vi "Test App Trigger Broadcast of Owned Process.vi"(8 "error in (no error)":errorcluster, 11 "Application Test in":refnum<class "Application Dev Test.lvclass">) -> (0 "error out":errorcluster, 3 "Application Test out":refnum<class "Application Dev Test.lvclass">)   [LabVIEW 2020, in "Application Dev Test.lvclass"]
uses:
  Application Dev Test.lvclass
  C:/Program Files (x86)/National Instruments/LabVIEW 2020/vi.lib/Astemes/LUnit/Test Case.lvclass
  source/Framework/Process/Process.lvclass
  source/Framework/Process/Process.lvclass/Process.ctl
  source/Framework/Application/Application.lvclass/Application.ctl
  <vilib>/Astemes/LUnit/Test Case.lvclass/Test Case.ctl
  <vilib>/Astemes/LUnit/LUnit Assertion Result.lvclass/LUnit Assertion Result.ctl
  <vilib>/Astemes/LUnit/LUnit Test Case Result.lvclass/LUnit Test Case Result.ctl
  <vilib>/Astemes/LUnit/LUnit Method Result.lvclass/LUnit Method Result.ctl
  source/Framework/Application/Private/Add Process to Map.vi
  source/Framework/Application/Private/Start Idle Processes if Running.vi
  source/Framework/Application/Private/Throw Error If Process Already in App.vi
  source/Framework/Process/Protected/Messaging/Enqueue Message.vi
  source/Framework/Process/Public/Lifecycle/Get Lifecycle State.vi
  source/Framework/Process/Protected/SubVIs/Set Context.vi
  source/Framework/Process/Private/SubVIs/Wait for finish.vi
  source/Framework/Process/Private/SubVIs/Set Lifecycle State.vi
  <vilib>/Astemes/LUnit/Palette/Fail.vi
  <vilib>/Astemes/LUnit/Palette/Pass.vi
  <vilib>/Astemes/LUnit/Set Assertion Type.vi
  source/Framework/Application/Public/Get Process.vi
  source/Framework/Process/Private/SubVIs/Handle Debug Data.vi
  <vilib>/Utility/error.llb/Clear Errors.vi
  source/Framework/Process/Public/Lifecycle/Leave Process Loop.vi
  <vilib>/Astemes/LUnit/Add test result.vi
  <vilib>/Astemes/LUnit/LUnit Write Passed.vi
  <vilib>/Astemes/LUnit/LUnit Write Message.vi
  <vilib>/Astemes/LUnit/LUnit Write Description.vi
  <vilib>/Astemes/LUnit/LUnit Write Assertion Type.vi
  source/Framework/Application/Private/Retrieve Process from App.vi
  source/Framework/Application/Private/Parse Process Name.vi
  source/Framework/Application/Private/Get Process from Map.vi
  source/Framework/Logging/Log Debug.vi
  <vilib>/AdvancedString/1D String Array to Delimited String.vi
  <vilib>/Utility/High Resolution Relative Seconds.vi
  <vilib>/Astemes/LUnit/LUnit Record Assertion Result.vi
  source/Framework/Process/Protected/Messaging/Request Message.vi
  <vilib>/AdvancedString/Delimited String to 1D String Array.vi
  <vilib>/Astemes/LUnit/LUnit Aggregate Assertion Results.vi
  source/Framework/Process/Private/SubVIs/Enqueue Request Message.vi
  <vilib>/Astemes/LUnit/Assertion Result/LUnit Read Status.vi
  <vilib>/Astemes/LUnit/LUnit Read Message.vi
  <vilib>/Astemes/LUnit/LUnit Read Description.vi
  <vilib>/Astemes/LUnit/Method Result/LUnit Merge Status.vi
  <vilib>/Astemes/LUnit/LUnit Concatenate result strings.vi
  source/Framework/Application/Application.lvclass
  C:/Git/astemes-triarc-framework/source/Framework/Process/Process.lvclass
  <vilib>/Utility/error.llb/Error Cluster From Error Code.vi
  source/Framework/Process/Public/Read Name.vi
  source/Framework/Process/Private/SubVIs/Wait for Response Message.vi
  <vilib>/Astemes/LUnit/LUnit Assertion Result.lvclass
  Application Dev Test.lvclass/Application Dev Test.ctl
  <vilib>/Astemes/LUnit/Test Case.lvclass
  source/Framework Test Suite/Support/Framework Test Support.lvlib
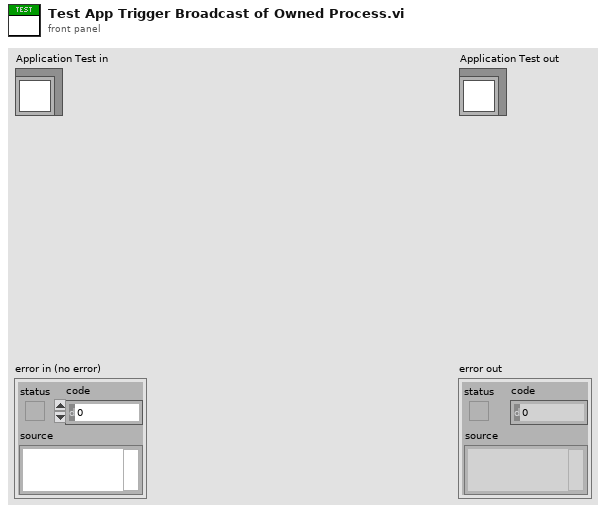
[diagram p1: front panel]
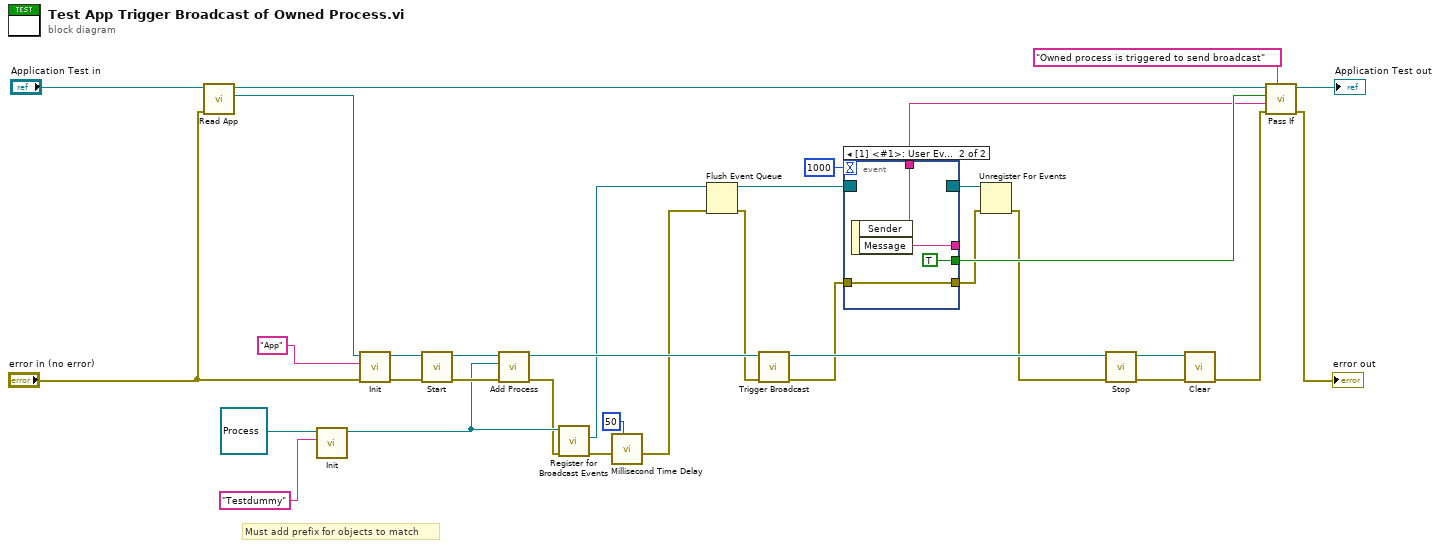
[diagram p0: block diagram]
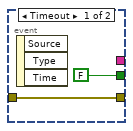
[diagram p2: hidden frame]
diagram:
  # "Must add prefix for objects to match"
  n1 = call "Read App.vi"("error in (no error)"="error in (no error)", "Application Test In"="Application Test in") -> ("App out"=w33:refnum<class "Application.lvclass">, "Application Test Out"=w34:refnum<class "Application Dev Test.lvclass">)  [unwired: 7 in, 1 out]
  n2 = call-dynamic "Init.vi"("Name"="Testdummy", "Process In"=refnum<class "Process.lvclass"> refnum ("Process.lvclass")) -> ("Process Out"=w21:refnum<class "Process.lvclass">)  [unwired: 8 in, 1 out]
  n3 = call-dynamic "Init.vi"("error in (no error)"="error in (no error)", "Name"="App", "Process In"=w33) -> ("error out"=w31:errorcluster, "Process Out"=w32:refnum<class "Application.lvclass">)  [unwired: 7 in]
  n4 = call "Start.vi"("error in (no error)"=w31, "Process In"=w32) -> ("error out"=w29:errorcluster, "Process Out"=w22:refnum<class "Application.lvclass">)  [unwired: 7 in, 1 out]
  n5 = call "Add Process.vi"("error in (no error)"=w29, "Process"=w21, "Application In"=w22) -> ("error out"=w20:errorcluster, "Application Out"=w19:refnum<class "Application.lvclass">)  [unwired: 7 in]
  n6 = call "Register for Broadcast Events.vi"("error in (no error)"=w20, "Process In"=w21) -> ("error out"=w5:errorcluster, "Event Registration Refnum Out"=w8:refnum<event-registration>)  [unwired: 7 in, 1 out]
  n7 = call "Millisecond Time Delay.vi"("milliseconds to wait"=u32 50, "error in (no error)"=w5) -> ("error out"=w4:errorcluster)  [unwired: 7 in]
  n8 = Flush Event Queue(0:w8, 3:w4) -> (8:w7:refnum<event-registration>, 11:w6:errorcluster)  [unwired: 4 in, 1 out]
  n9 = call "Trigger Broadcast.vi"("error in (no error)"=w6, "Process in"=w19) -> ("error out"=w10:errorcluster, "Process out"=w18:refnum<class "Application.lvclass">)  [unwired: 8 in]
  n10 = event shown="[1] <#1>: User Event" {
    selector: w7 -> [_ _]
    dyn-events: [_ _] -> w17
    timeout: 1000 -> [_ _]
    tunnel: [FALSE TRUE] -> w15
    tunnel: [w35 w39] -> w2
    tunnel: w10 -> [w35 w39]
    tunnel: [_ w38] -> w9
    tunnel: [_ w37] -> _
    event Timeout {
      n11 = event-data() -> ()  [unwired: 1 in, 3 out]
    }
    event User Event {
      n12 = event-data() -> ("Sender"=w38:string, "Message"=w37:string)  [unwired: 1 in]
    }
  }
  n13 = Unregister For Events(event registration refnum=w17, error in=w2) -> (error out=w1:errorcluster)
  n14 = call "Stop.vi"("error in (no error)"=w1, "Process In"=w18) -> ("error out"=w27:errorcluster, "Process Out"=w30:refnum<class "Application.lvclass">)  [unwired: 7 in, 1 out]
  n15 = call-dynamic "Clear.vi"("error in (no error)"=w27, "Application In"=w30) -> ("error out"=w14:errorcluster)  [unwired: 9 in]
  n16 = call <vilib>:"Pass If.vi"("Description"="Owned process is triggered to send broadcast", "error in (no error)"=w14, "Message"=w9, "Pass?"=w15, "LUnit Test Case In"=w34) -> ("error out"=→"error out":errorcluster, "LUnit Test Case Out"=→"Application Test out":refnum<class "Application Dev Test.lvclass">)  [unwired: 5 in]
